vi "Channel Page.vi"(8 "error in (no error)":errorcluster, 11 "Node Ptr":T3 format="%.0x") -> (0 "error out":errorcluster)   [LabVIEW 2011, in "PXIe-433x Custom Device.lvlib"]
uses:
  PXIe-433x Custom Device.lvlib
  <vilib>/NI Veristand/Custom Device API/Custom Device Item Ref.ctl
  Channel #.ctl
  Sensor Type.ctl
  Generic Bridge Information.ctl
  Strain Information.ctl
  Strain Bridge Information.ctl
  Force Scaling Information.ctl
  Pressure Scaling Information.ctl
  Torque Scaling Information.ctl
  Global.vi
  <vilib>/NI Veristand/Custom Device API/Get Item Property (U16).vi
  <vilib>/NI Veristand/Custom Device API/Get Item Property (Variant).vi
  <vilib>/NI Veristand/Custom Device API/Set Item Property (Variant).vi
  <vilib>/NI Veristand/Custom Device API/Set Item Property (Double).vi
  <vilib>/NI Veristand/Custom Device API/Set Item Property (U16).vi
  <vilib>/NI Veristand/Custom Device API/Custom Device API.lvlib
panel:
  in  "Sensor Type":T1
  in  "Channel #":T2
  in  "Header":cluster{"Section Name":string}={"Section Name"="Input Channel Settings"}
  in  "Description":string
  in  "Name":string
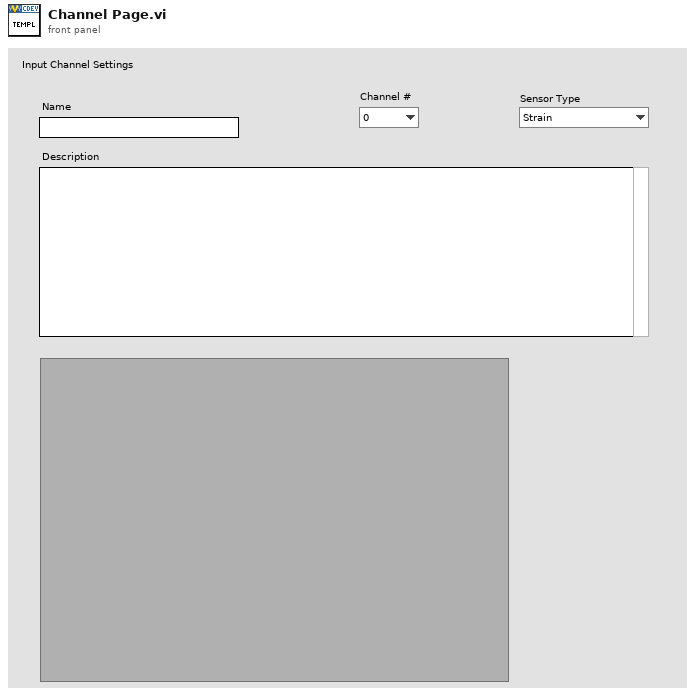
[diagram p1: front panel]
types:
  T1 = typedef "PXIe-433x Custom Device.lvlib/Sensor Type.ctl" = enum16{"Strain", "Force", "Pressure", "Torque"}
  T2 = typedef "PXIe-433x Custom Device.lvlib/Channel #.ctl" = enum16{"0", "1", "2", "3", "4", "5", "6", "7"}
  T3 = typedef "Custom Device API.lvlib/Custom Device Item Ref.ctl" = u64
  T4 = typedef "PXIe-433x Custom Device.lvlib/Board Info for checking settings.ctl" = cluster{"Present?":bool, "Created by CD code?":bool, "Resource Name":string}
  T5 = typedef "Custom Device API.lvlib/Custom Device Item Info.ctl" = cluster{"Name":string, "Is Channel":bool, "GUID":string}
  T6 = typedef "PXIe-433x Custom Device.lvlib/Generic Bridge Information.ctl" = cluster{"bridge configuration":i32, "voltage excitation source":i32, "voltage excitation value":dbl, "nominal bridge resistance":dbl}
  T7 = typedef "PXIe-433x Custom Device.lvlib/Strain Information.ctl" = cluster{"gage factor":dbl, "nominal gage resistance":dbl, "poisson ratio":dbl}
  T8 = typedef "PXIe-433x Custom Device.lvlib/Strain Bridge Information.ctl" = cluster{"strain configuration":i32, "lead wire resistance":dbl, "initial bridge voltage":dbl, "voltage excitation source":i32, "voltage excitation value":dbl}
  T9 = typedef "Custom Device API.lvlib/Custom Device Commands.ctl" = enum16{"Default", "Item renamed", "Shutdown", "Dynamic button pressed"}
  T10 = typedef "PXIe-433x Custom Device.lvlib/Force Scaling Information.ctl" = cluster{"first electrical value":dbl, "second electrical value":dbl, "electrical units":i32, "first physical value":dbl, "second physical value":dbl, "physical units":i32}
  T11 = typedef "PXIe-433x Custom Device.lvlib/Pressure Scaling Information.ctl" = cluster{"first electrical value":dbl, "second electrical value":dbl, "electrical units":i32, "first physical value":dbl, "second physical value":dbl, "physical units":i32}
  T12 = typedef "PXIe-433x Custom Device.lvlib/Torque Scaling Information.ctl" = cluster{"first electrical value":dbl, "second electrical value":dbl, "electrical units":i32, "first physical value":dbl, "second physical value":dbl, "physical units":i32}
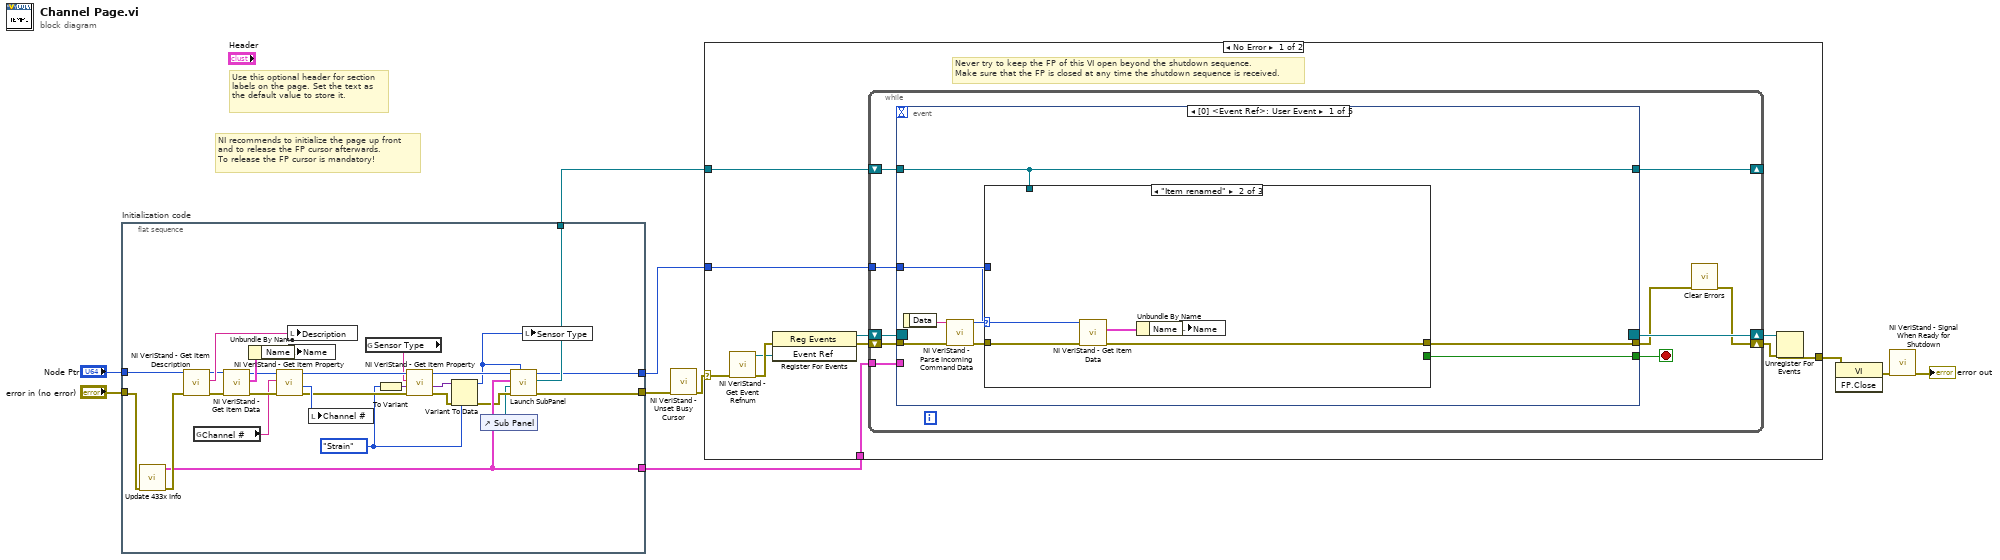
[diagram p0: block diagram]
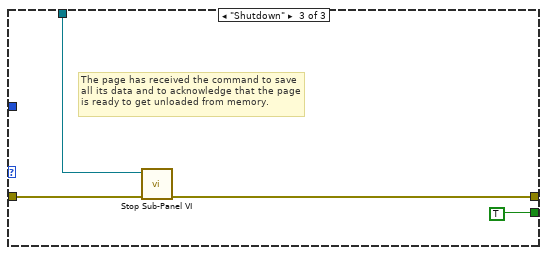
[diagram p3: hidden frame]
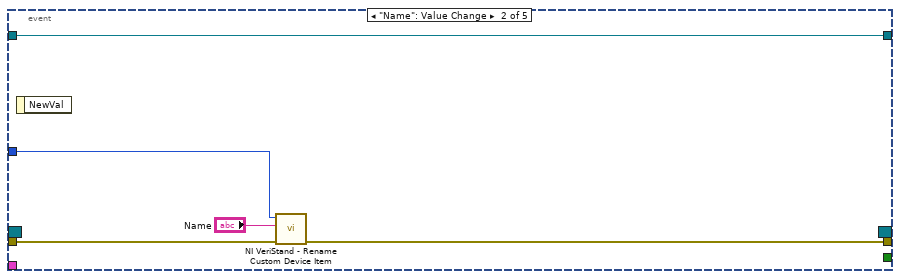
[diagram p4: hidden frame]
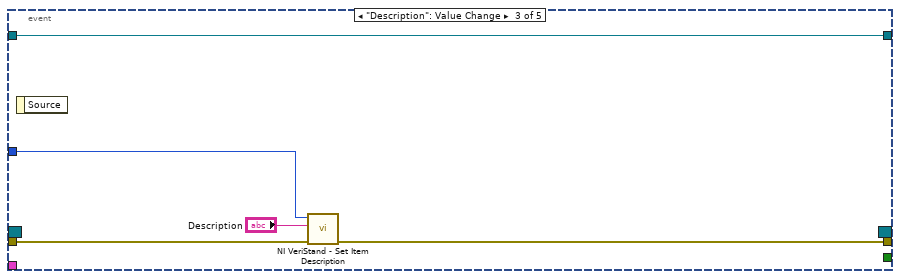
[diagram p5: hidden frame]
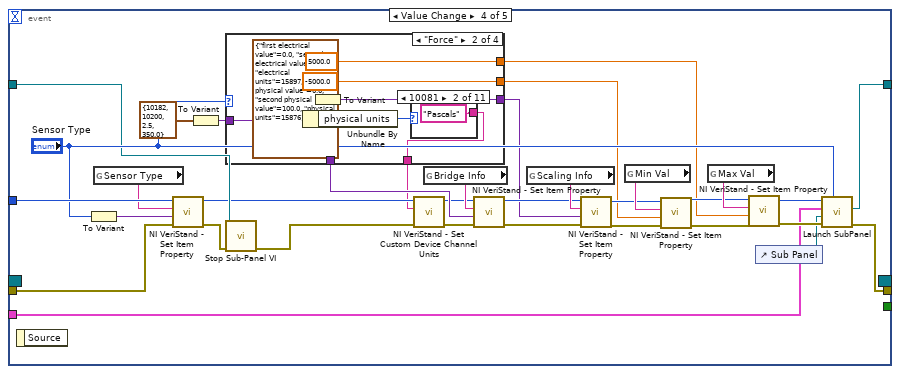
[diagram p6: hidden frame]
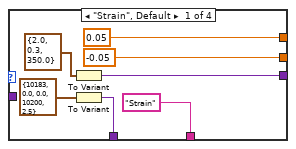
[diagram p7: hidden frame]
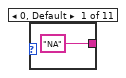
[diagram p8: hidden frame]
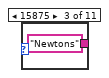
[diagram p9: hidden frame]
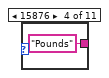
[diagram p10: hidden frame]
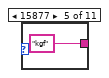
[diagram p11: hidden frame]
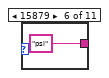
[diagram p12: hidden frame]
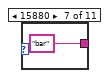
[diagram p13: hidden frame]
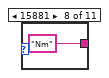
[diagram p14: hidden frame]
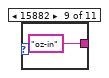
[diagram p15: hidden frame]
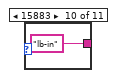
[diagram p16: hidden frame]
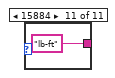
[diagram p17: hidden frame]
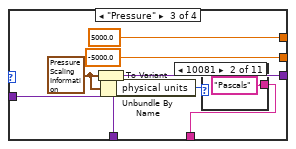
[diagram p18: hidden frame]
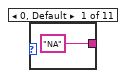
[diagram p19: hidden frame]
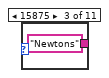
[diagram p20: hidden frame]
diagram:
  # "Use this optional header for section labels on the page. Set the text as the default value to store it."
  # "NI recommends to initialize the page up front\nand to release the FP cursor afterwards.\nTo release the FP cursor is mandatory!"
  n1 = flat-sequence "Initialization code" {
    tunnel: "error in (no error)" -> [w16]
    tunnel: "Node Ptr" -> [w37]
    tunnel: [w12] -> w7
    tunnel: [w19] -> w4
    tunnel: [w17] -> w2
    tunnel: [w14] -> w1
    frame #0 {
      w21 = Sensor_Type."Strain" ("Sensor Type")
      n2 = call "Update 433x Info.vi"("error in (no error)"=w16) -> ("error IO"=w15:errorcluster, "Board Info for checking"=w14:T4)  [unwired: 9 in]
      n3 = call <vilib>:"NI VeriStand - Get Item Description.vi"("error in (no error)"=w15, "Item Ref in"=w37) -> ("error out"=w35:errorcluster, "Description"=w36:string, "Item Ref out"=w34:T3)  [unwired: 7 out]
      n4 = global read "Global.vi" "Channel #"() -> (w29:string)
      n5 = call <vilib>:"NI VeriStand - Get Item Data.vi"("error in (no error)"=w35, "Item Ref in"=w34) -> ("error out"=w31:errorcluster, "Item Info"=w33:T5, "Item Ref out"=w30:T3)  [unwired: 7 out]
      n6 = Unbundle By Name(w33) -> ("Name"=w32:string)
      n7 = call-poly <vilib>:"NI VeriStand - Get Item Property.vi"("error in (no error)"=w31, "Property Name"=w29, "Item Ref in"=w30) -> ("error out"=w27:errorcluster, "Value"=w28:u16, "Item Ref out"=w26:T3)  [unwired: 5 in, 1 out]
      n8 = local write "Description"(w36) -> ()
      n9 = local write "Name"(w32) -> ()
      n10 = local write "Channel #"(w28) -> ()
      n11 = global read "Global.vi" "Sensor Type"() -> (w25:string)
      n12 = To Variant(anything=w21) -> (Variant=w24:variant)
      n13 = call-poly <vilib>:"NI VeriStand - Get Item Property.vi"("error in (no error)"=w27, "Default Value"=w24, "Property Name"=w25, "Item Ref in"=w26) -> ("error out"=w22:errorcluster, "Value"=w23:variant, "Item Ref out"=w20:T3)  [unwired: 4 in, 1 out]
      n14 = Variant To Data(error in=w22, type=w21, Variant=w23) -> (data=w18:T1, error out=w13:errorcluster)
      n15 = control-ref of="Sub Panel"() -> (w11:refnum<vi>)
      n16 = call "Launch SubPanel.vi"("Sensor Type"=w18, "error in"=w13, "Sub Panel"=w11, "Board Info for checking"=w14, "Item Ref in"=w20) -> ("error out"=w12:errorcluster, "VI Refnum"=w19:refnum<vi>, "Item Ref out"=w17:T3)  [unwired: 4 in]
      n17 = local write "Sensor Type"(w18) -> ()
    }
  }
  n18 = call <vilib>:"NI VeriStand - Unset Busy Cursor.vi"("error in (no error)"=w7) -> ("error out"=w6:errorcluster)  [unwired: 10 out]
  n19 = case shown="No Error" w6 {
    selector: w6 -> [w40 w216]
    tunnel: [w45 w214] -> w10
    tunnel: w2 -> [w41 _]
    tunnel: w4 -> [w39 _]
    tunnel: w1 -> [w38 _]
    frame No Error {
      # "Never try to keep the FP of this VI open beyond the shutdown sequence.\nMake sure that the FP is closed at any time the shutdown sequence is received."
      n20 = call <vilib>:"NI VeriStand - Get Event Refnum.vi"("error in (no error)"=w40) -> ("error out"=w48:errorcluster, "Event Ref"=w44:refnum<user-event>)  [unwired: 9 out]
      n21 = register-events(error in=w48, w44) -> (reference out=w42:refnum<event-registration>, error out=w43:errorcluster)  [unwired: 1 in]
      n22 = while {
        tunnel: w41 -> [w54]
        shift-right: [w53] -> w46
        shift-left: w43 -> [w57]
        shift-right: [w58] -> w47
        shift-left: w42 -> [w56]
        shift-right: [w51] -> _
        shift-left: w39 -> [w52]
        tunnel: w38 -> [w50]
        stop <- w55 stop-if-true
        n23 = event shown="[0] <Event Ref>: User Event" {
          selector: w56 -> [_ _ _ _ _]
          dyn-events: [_ _ _ _ _] -> w58
          timeout: _ -> [_ _ _ _ _]
          tunnel: w57 -> [w66 w81 w85 w117 w198]
          tunnel: [w62 _ _ _ _] -> w55
          tunnel: [w61 w80 w84 w93 w184] -> w49
          tunnel: w54 -> [w60 w79 w86 w120 w197]
          tunnel: w52 -> [w59 w77 w82 w105 w182]
          tunnel: [w59 w77 w82 w116 w182] -> w51
          tunnel: w50 -> [_ _ _ w94 _]
          event User Event {
            n24 = event-data() -> ("Data"=w65:string)  [unwired: 1 out]
            n25 = call <vilib>:"NI VeriStand - Parse Incoming Command Data.vi"("error in (no error)"=w66, "Incoming data"=w65) -> ("error out"=w64:errorcluster, "Action"=w63:T9)  [unwired: 8 out]
            n26 = case shown="\"Item renamed\"" w63 {
              tunnel: w64 -> [w67 w72 w75]
              tunnel: [_ _ TRUE] -> w62
              tunnel: [w67 w69 w74] -> w61
              tunnel: w60 -> [_ w71 _]
              tunnel: w59 -> [_ _ w73]
              frame "Default", Default {
              }
              frame "Item renamed" {
                n27 = call <vilib>:"NI VeriStand - Get Item Data.vi"("error in (no error)"=w72, "Item Ref in"=w71) -> ("error out"=w69:errorcluster, "Item Info"=w70:T5)  [unwired: 8 out]
                n28 = Unbundle By Name(w70) -> ("Name"=w68:string)
                n29 = local write "Name"(w68) -> ()
              }
              frame "Shutdown" {
                # "The page has received the command to save all its data and to acknowledge that the page is ready to get unloaded from memory."
                n30 = call "Stop Sub-Panel VI.vi"("error in (no error) 2"=w75, "reference"=w73) -> ("error IO"=w74:errorcluster)  [unwired: 9 in]
              }
            }
          }
          event "Name": Value Change {
            n31 = event-data() -> ()  [unwired: 2 out]
            n32 = call <vilib>:"NI VeriStand - Rename Custom Device Item.vi"("error in (no error)"=w81, "New Name"="Name", "Item Ref in"=w79) -> ("error out"=w80:errorcluster)  [unwired: 8 out]
          }
          event "Description": Value Change {
            n33 = event-data() -> ()  [unwired: 2 out]
            n34 = call <vilib>:"NI VeriStand - Set Item Description.vi"("error in (no error)"=w85, "Description"="Description", "Item Ref in"=w86) -> ("error out"=w84:errorcluster)  [unwired: 8 out]
          }
          event Value Change {
            n35 = event-data() -> ()  [unwired: 2 out]
            n36 = To Variant(anything="Sensor Type") -> (Variant=w118:variant)
            n37 = global read "Global.vi" "Sensor Type"() -> (w119:string)
            n38 = call-poly <vilib>:"NI VeriStand - Set Item Property.vi"("error in (no error)"=w117, "Value"=w118, "Property Name"=w119, "Item Ref in"=w120) -> ("error out"=w106:errorcluster, "Item Ref out"=w89:T3)  [unwired: 5 in, 1 out]
            n39 = To Variant(anything=T6 {"bridge configuration"=10182, "voltage excitation source"=10200, "voltage excitation value"=2.5, "nominal bridge resistance"=350.0} ("bridge information")) -> (Variant=w107:variant)
            n40 = case shown="\"Force\"" "Sensor Type" {
              tunnel: [w126 w133 w151 w169] -> w109
              tunnel: [w127 w134 w152 w170] -> w110
              tunnel: w107 -> [_ w133 w151 w169]
              tunnel: [-0.05 -5000.0 -5000.0 -5000.0] -> w96
              tunnel: [0.05 5000.0 5000.0 5000.0] -> w95
              tunnel: ["Strain" ("Units") w128 w146 w164] -> w87
              frame "Strain", Default {
                n41 = To Variant(anything=T7 {"gage factor"=2.0, "nominal gage resistance"=0.3, "poisson ratio"=350.0} ("strain gage information")) -> (Variant=w127:variant)
                n42 = To Variant(anything=T8 {"strain configuration"=10183, "lead wire resistance"=0.0, "initial bridge voltage"=0.0, "voltage excitation source"=10200, "voltage excitation value"=2.5} ("bridge information")) -> (Variant=w126:variant)
              }
              frame "Force" {
                w130 = T10 {"first electrical value"=0.0, "second electrical value"=2.0, "electrical units"=15897, "first physical value"=0.0, "second physical value"=100.0, "physical units"=15876} ("scaling information")
                n43 = Unbundle By Name(w130) -> ("physical units"=w129:i32)
                n44 = To Variant(anything=w130) -> (Variant=w134:variant)
                n45 = case shown="10081" w129 {
                  tunnel: ["NA" "Pascals" "Newtons" "Pounds" "kgf" "psi" "bar" "Nm" "oz-in" "lb-in" "lb-ft"] -> w128
                  frame 0, Default {
                  }
                  frame 10081 {
                  }
                  frame 15875 {
                  }
                  frame 15876 {
                  }
                  frame 15877 {
                  }
                  frame 15879 {
                  }
                  frame 15880 {
                  }
                  frame 15881 {
                  }
                  frame 15882 {
                  }
                  frame 15883 {
                  }
                  frame 15884 {
                  }
                }
              }
              frame "Pressure" {
                w148 = T11 {"first electrical value"=0.0, "second electrical value"=2.0, "electrical units"=15897, "first physical value"=0.0, "second physical value"=100.0, "physical units"=15879} ("scaling information")
                n46 = To Variant(anything=w148) -> (Variant=w152:variant)
                n47 = Unbundle By Name(w148) -> ("physical units"=w147:i32)
                n48 = case shown="10081" w147 {
                  tunnel: ["NA" "Pascals" "Newtons" "Pounds" "kgf" "psi" "bar" "Nm" "oz-in" "lb-in" "lb-ft"] -> w146
                  frame 0, Default {
                  }
                  frame 10081 {
                  }
                  frame 15875 {
                  }
                  frame 15876 {
                  }
                  frame 15877 {
                  }
                  frame 15879 {
                  }
                  frame 15880 {
                  }
                  frame 15881 {
                  }
                  frame 15882 {
                  }
                  frame 15883 {
                  }
                  frame 15884 {
                  }
                }
              }
              frame "Torque" {
                w166 = T12 {"first electrical value"=0.0, "second electrical value"=2.0, "electrical units"=15897, "first physical value"=0.0, "second physical value"=100.0, "physical units"=15883} ("scaling information")
                n49 = Unbundle By Name(w166) -> ("physical units"=w165:i32)
                n50 = To Variant(anything=w166) -> (Variant=w170:variant)
                n51 = case shown="10081" w165 {
                  tunnel: ["NA" "Pascals" "Newtons" "Pounds" "kgf" "psi" "bar" "Nm" "oz-in" "lb-in" "lb-ft"] -> w164
                  frame 0, Default {
                  }
                  frame 10081 {
                  }
                  frame 15875 {
                  }
                  frame 15876 {
                  }
                  frame 15877 {
                  }
                  frame 15879 {
                  }
                  frame 15880 {
                  }
                  frame 15881 {
                  }
                  frame 15882 {
                  }
                  frame 15883 {
                  }
                  frame 15884 {
                  }
                }
              }
            }
            n52 = call "Stop Sub-Panel VI.vi"("error in (no error) 2"=w106, "reference"=w105) -> ("error IO"=w91:errorcluster)  [unwired: 9 in]
            n53 = call <vilib>:"NI VeriStand - Set Custom Device Channel Units.vi"("error in (no error)"=w91, "Units"=w87, "Channel Ref in"=w89) -> ("error out"=w90:errorcluster, "Channel Ref out"=w88:T3)  [unwired: 7 in]
            n54 = global read "Global.vi" "Bridge Info"() -> (w115:string)
            n55 = call-poly <vilib>:"NI VeriStand - Set Item Property.vi"("error in (no error)"=w90, "Value"=w109, "Property Name"=w115, "Item Ref in"=w88) -> ("error out"=w112:errorcluster, "Item Ref out"=w113:T3)  [unwired: 5 in, 1 out]
            n56 = global read "Global.vi" "Scaling Info"() -> (w114:string)
            n57 = call-poly <vilib>:"NI VeriStand - Set Item Property.vi"("error in (no error)"=w112, "Value"=w110, "Property Name"=w114, "Item Ref in"=w113) -> ("error out"=w102:errorcluster, "Item Ref out"=w97:T3)  [unwired: 5 in, 1 out]
            n58 = global read "Global.vi" "Min Val"() -> (w104:string)
            n59 = call-poly <vilib>:"NI VeriStand - Set Item Property.vi"("error in (no error)"=w102, "Value"=w96, "Property Name"=w104, "Item Ref in"=w97) -> ("error out"=w101:errorcluster, "Item Ref out"=w98:T3)  [unwired: 5 in, 1 out]
            n60 = global read "Global.vi" "Max Val"() -> (w103:string)
            n61 = call-poly <vilib>:"NI VeriStand - Set Item Property.vi"("error in (no error)"=w101, "Value"=w95, "Property Name"=w103, "Item Ref in"=w98) -> ("error out"=w100:errorcluster, "Item Ref out"=w99:T3)  [unwired: 5 in, 1 out]
            n62 = control-ref of="Sub Panel"() -> (w92:refnum<vi>)
            n63 = call "Launch SubPanel.vi"("Sensor Type"="Sensor Type", "error in"=w100, "Sub Panel"=w92, "Board Info for checking"=w94, "Item Ref in"=w99) -> ("error out"=w93:errorcluster, "VI Refnum"=w116:refnum<vi>)  [unwired: 4 in, 1 out]
          }
          event Value Change {
            n64 = event-data() -> ("OldVal"=w183:T2)  [unwired: 1 out]
            n65 = call <vilib>:"NI VeriStand - Get Item Parent.vi"("error in (no error)"=w198, "Item Ref in"=w197) -> ("error out"=w196:errorcluster, "Parent Ref"=w195:T3, "Item Ref out"=w187:T3)  [unwired: 6 in, 1 out]
            n66 = call <vilib>:"NI VeriStand - Get Item Children.vi"("error in (no error)"=w196, "Item Ref in"=w195) -> ("error out"=w193:errorcluster, "Child Refs"=w194:T3[])  [unwired: 6 in, 2 out]
            n67 = for {
              tunnel: w194 -> [w210] mode=indexing
              shift-right: [w212] -> w188
              shift-left: w193 -> [w213]
              tunnel: [w209] -> w192 mode=indexing
              n68 = global read "Global.vi" "Channel #"() -> (w211:string)
              n69 = call-poly <vilib>:"NI VeriStand - Get Item Property.vi"("error in (no error)"=w213, "Property Name"=w211, "Item Ref in"=w210) -> ("error out"=w212:errorcluster, "Value"=w209:u16)  [unwired: 5 in, 2 out]
            }
            n70 = global read "Global.vi" "Channel #"() -> (w186:string)
            n71 = Search 1D Array(1D array=w192, element="Channel #") -> (index of element=w191:i32)  [unwired: 1 in]
            n72 = Equal?(x=w191, y=-1) -> (x = y?=w189:bool)
            n73 = case shown="True" w189 {
              tunnel: w188 -> [w200 w208]
              tunnel: w187 -> [_ w207]
              tunnel: w186 -> [_ w203]
              tunnel: "Channel #" -> [_ w202]
              tunnel: [w200 w205] -> w184
              tunnel: w183 -> [w201 _]
              frame False {
                n74 = local write "Channel #"(w201) -> ()
                n75 = One Button Dialog(message="Channel Already Exists") -> ()  [unwired: 1 in, 1 out]
              }
              frame True {
                n76 = call "Change Name.vi"("error in (no error)"=w208, "New #"=w202, "Node Ptr"=w207) -> ("error out"=w206:errorcluster, "Node Ptr out"=w204:T3)  [unwired: 7 in]
                n77 = call-poly <vilib>:"NI VeriStand - Set Item Property.vi"("error in (no error)"=w206, "Value"=w202, "Property Name"=w203, "Item Ref in"=w204) -> ("error out"=w205:errorcluster)  [unwired: 5 in, 2 out]
              }
            }
          }
        }
        n78 = call <vilib>:"Clear Errors.vi"("error in (no error)"=w49) -> ("error out"=w53:errorcluster)  [unwired: 6 out]
      }
      n79 = Unregister For Events(event registration refnum=w47, error in=w46) -> (error out=w45:errorcluster)
    }
    frame Error {
      n80 = call <vilib>:"Simple Error Handler.vi"("error in (no error)"=w216) -> ("error out"=w215:errorcluster)  [unwired: 1 in, 7 out]
      n81 = call <vilib>:"Clear Errors.vi"("error in (no error)"=w215) -> ("error out"=w214:errorcluster)  [unwired: 6 out]
    }
  }
  n82 = invoke class="VI" method="FP.Close"(error in=w10) -> (error out=w9:errorcluster)  [unwired: 2 in, 2 out]
  n83 = call <vilib>:"NI VeriStand - Signal When Ready for Shutdown.vi"("error in (no error)"=w9) -> ("error out"=→"error out":errorcluster)  [unwired: 10 out]
